vi "UT_LokiHandler_Main.vi"(8 "error in (no error)":errorcluster) -> (0 "error out":errorcluster)   [LabVIEW 2017, in "UT_LokiHandler.lvlib"]
uses:
  UT_LokiHandler.lvlib
  <vilib>/addons/_JKI Toolkits/Caraya/classes/Test/Test.lvclass
panel:
  # "Connector Pane"
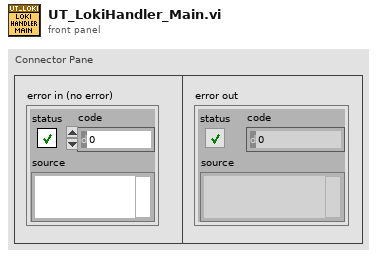
[diagram p1: front panel]
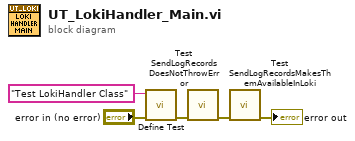
[diagram p0: block diagram]
diagram:
  n1 = call <vilib>:"Define Test.vi"("error in (no error)"="error in (no error)", "Label (VI Title)"="Test LokiHandler Class") -> ("error out"=w3:errorcluster)  [unwired: 8 in, 1 out]
  n2 = call "Test SendLogRecordsDoesNotThrowError.vi"("error in (no error)"=w3) -> ("error out"=w5:errorcluster)  [unwired: 10 in]
  n3 = call "Test SendLogRecordsMakesThemAvailableInLoki.vi"("error in (no error)"=w5) -> ("error out"=→"error out":errorcluster)  [unwired: 10 in]
